vi "StateMachineWithIdleCase.vi"() -> ()   [LabVIEW 2020]
uses:
  States.ctl
panel:
  in  "stop":bool
  in  "Process2":bool
  in  "Process1":bool
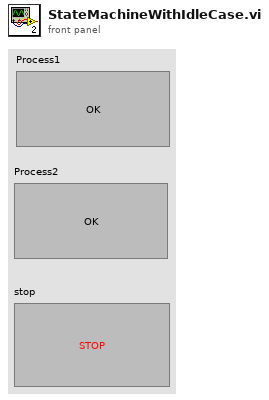
[diagram p1: front panel]
types:
  T1 = typedef "States.ctl" = enum16{"Idle", "Initialize", "IncrementNumber", "UpdateUI", "Process2", "Exit"}
  T2 = typedef "States.ctl" = enum16{"Idle", "Initialize", "Process1", "Process2", "Exit"}
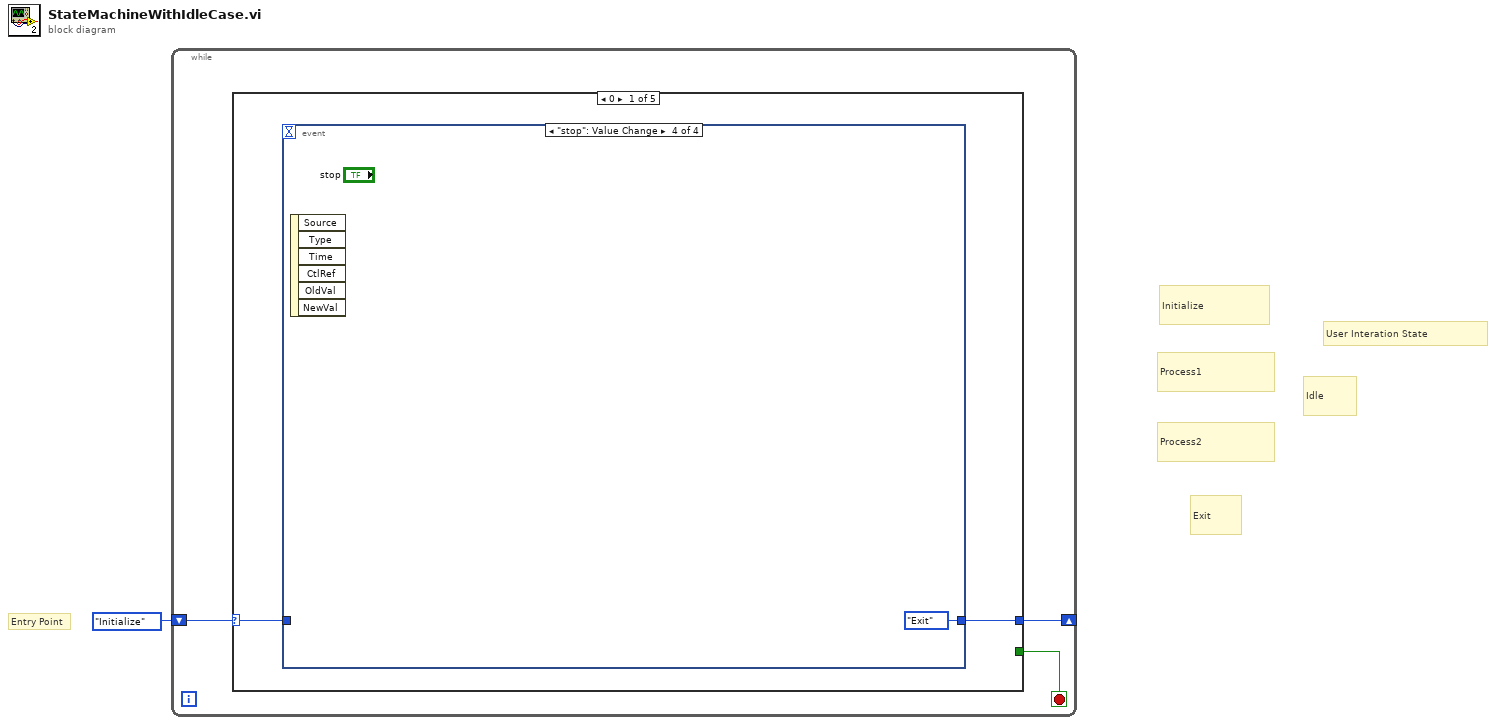
[diagram p0: block diagram]
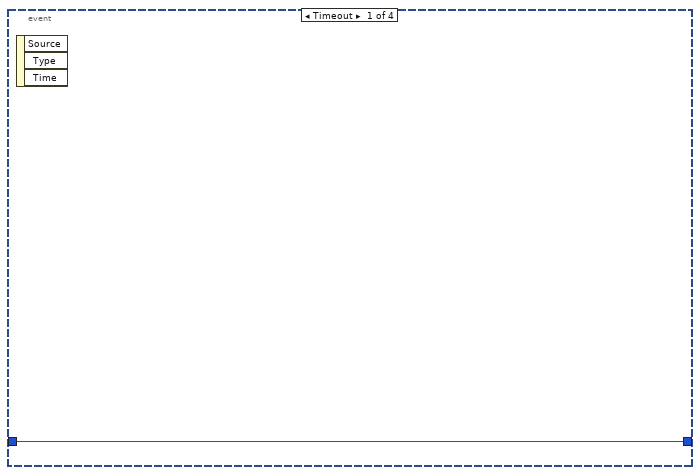
[diagram p2: hidden frame]
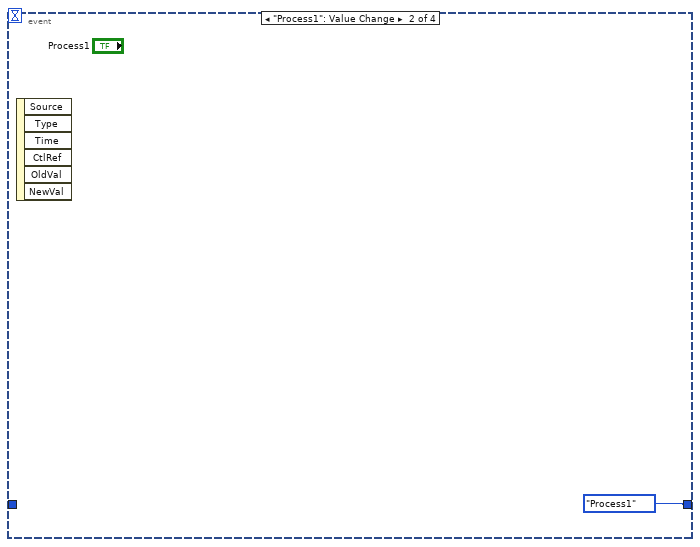
[diagram p3: hidden frame]
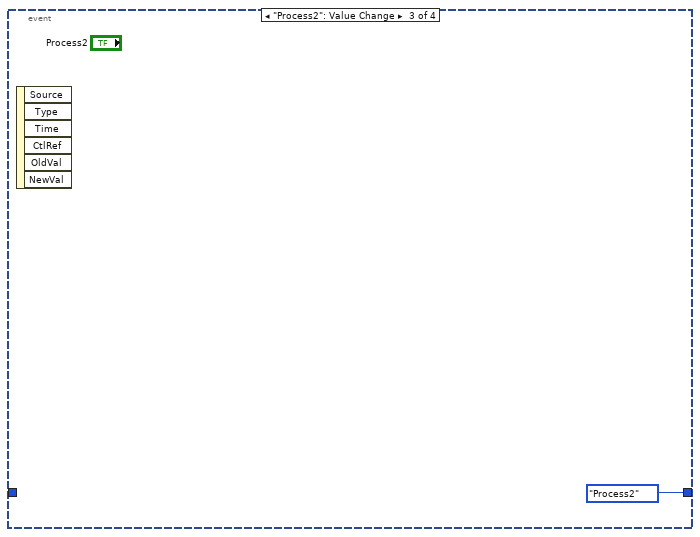
[diagram p4: hidden frame]
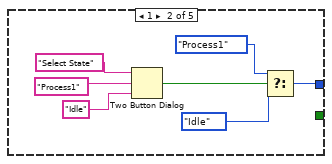
[diagram p5: hidden frame]
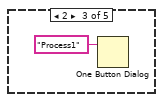
[diagram p6: hidden frame]
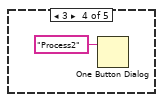
[diagram p7: hidden frame]
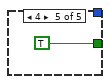
[diagram p8: hidden frame]
diagram:
  # "User Interation State"
  # "Entry Point"
  # "Idle"
  # "Exit"
  # "Process2"
  # "Process1"
  # "Initialize"
  n1 = while {
    shift-right: [w3] -> _
    shift-left: States."Initialize" -> [w4]
    stop <- w2 stop-if-true
    n2 = case shown="0" w4 {
      selector: w4 -> [w6 _ _ _ _]
      tunnel: [w5 w11 _ _ _] -> w3
      tunnel: [_ _ _ _ TRUE] -> w2
      frame 0 {
        n3 = event shown="[3] \"stop\": Value Change" {
          selector: _ -> [_ _ _ _]
          dyn-events: _ -> [_ _ _ _]
          timeout: _ -> [_ _ _ _]
          tunnel: w6 -> [w7 _ _ _]
          tunnel: [w7 States."Process1" States."Process2" States."Exit"] -> w5
          event Timeout {
            n4 = event-data() -> ()  [unwired: 1 in, 3 out]
          }
          event "Process1": Value Change {
            n5 = event-data() -> ()  [unwired: 1 in, 6 out]
          }
          event "Process2": Value Change {
            n6 = event-data() -> ()  [unwired: 1 in, 6 out]
          }
          event "stop": Value Change {
            n7 = event-data() -> ()  [unwired: 1 in, 6 out]
          }
        }
      }
      frame 1 {
        n8 = Two Button Dialog(message="Select State", 1:"Idle" ("message"), 2:"Process1" ("message")) -> (T button?=w14:bool)
        n9 = Select(t=States."Process1", s=w14, f=States."Idle") -> (s? t:f=w11:u16)
      }
      frame 2 {
        n10 = One Button Dialog(message="Process1") -> ()  [unwired: 1 in, 1 out]
      }
      frame 3 {
        n11 = One Button Dialog(message="Process2") -> ()  [unwired: 1 in, 1 out]
      }
      frame 4 {
      }
    }
  }
